vi "Rejestracja_konfiguracja.vi"(8 "error in (no error)":errorcluster, 11 "WolnaIn":T4={"WolnaStart"=FALSE, "WolnaPrzeglad"=FALSE, "Okres"=0.5, "Czas max"=120.0, "WolnaKonfiguracja"=FALSE, "Rej.1"={"Typ rejestracji"=enum."Wprost", "Kanały"=[1], "Opis"="Rej.X", "Aktywny"=FALSE, "Wolna Wykr num"=0}, "Rej.2"={"Typ rejestracji"=enum."Wprost", "Kanały"=[1], "Opis"="Rej.X", "Aktywny"=FALSE, "Wolna Wykr num"=0}, "Rej.3"={"Typ rejestracji"=enum."Wprost", "Kanały"=[1], "Opis"="Rej.X", "Aktywny"=FALSE, "Wolna Wykr num"=0}, "Rej.4"={"Typ rejestracji"=enum."Wprost", "Kanały"=[1], "Opis"="Rej.X", "Aktywny"=FALSE, "Wolna Wykr num"=0}, "Rej.5"={"Typ rejestracji"=enum."Wprost", "Kanały"=[1], "Opis"="Rej.X", "Aktywny"=FALSE, "Wolna Wykr num"=0}, "Rej.6"={"Typ rejestracji"=enum."Wprost", "Kanały"=[1], "Opis"="Rej.X", "Aktywny"=FALSE, "Wolna Wykr num"=0}, "Rej.7"={"Typ rejestracji"=enum."Wprost", "Kanały"=[1], "Opis"="Rej.X", "Aktywny"=FALSE, "Wolna Wykr num"=0}, "Rej.8"={"Typ rejestracji"=enum."Wprost", "Kanały"=[1], "Opis"="Rej.X", "Aktywny"=FALSE, "Wolna Wykr num"=0}} {"Rej.8"."Wolna Wykr num" items=["Brak", "Wykres 1", "Wykres 2", "Wykres 3", "Wykres 4"]; "Rej.7"."Wolna Wykr num" items=["Brak", "Wykres 1", "Wykres 2", "Wykres 3", "Wykres 4"]; "Rej.6"."Wolna Wykr num" items=["Brak", "Wykres 1", "Wykres 2", "Wykres 3", "Wykres 4"]; "Rej.5"."Wolna Wykr num" items=["Brak", "Wykres 1", "Wykres 2", "Wykres 3", "Wykres 4"]; "Rej.4"."Wolna Wykr num" items=["Brak", "Wykres 1", "Wykres 2", "Wykres 3", "Wykres 4"]; "Rej.3"."Wolna Wykr num" items=["Brak", "Wykres 1", "Wykres 2", "Wykres 3", "Wykres 4"]; "Rej.2"."Wolna Wykr num" items=["Brak", "Wykres 1", "Wykres 2", "Wykres 3", "Wykres 4"]; "Rej.1"."Wolna Wykr num" items=["Brak", "Wykres 1", "Wykres 2", "Wykres 3", "Wykres 4"]}) -> (0 "error out":errorcluster, 3 "WolnaOut":T4={"WolnaStart"=FALSE, "WolnaPrzeglad"=FALSE, "Okres"=0.5, "Czas max"=120.0, "WolnaKonfiguracja"=FALSE, "Rej.1"={"Typ rejestracji"=enum."Wprost", "Kanały"=[1], "Opis"="Rej.X", "Aktywny"=FALSE, "Wolna Wykr num"=0}, "Rej.2"={"Typ rejestracji"=enum."Wprost", "Kanały"=[1], "Opis"="Rej.X", "Aktywny"=FALSE, "Wolna Wykr num"=0}, "Rej.3"={"Typ rejestracji"=enum."Wprost", "Kanały"=[1], "Opis"="Rej.X", "Aktywny"=FALSE, "Wolna Wykr num"=0}, "Rej.4"={"Typ rejestracji"=enum."Wprost", "Kanały"=[1], "Opis"="Rej.X", "Aktywny"=FALSE, "Wolna Wykr num"=0}, "Rej.5"={"Typ rejestracji"=enum."Wprost", "Kanały"=[1], "Opis"="Rej.X", "Aktywny"=FALSE, "Wolna Wykr num"=0}, "Rej.6"={"Typ rejestracji"=enum."Wprost", "Kanały"=[1], "Opis"="Rej.X", "Aktywny"=FALSE, "Wolna Wykr num"=0}, "Rej.7"={"Typ rejestracji"=enum."Wprost", "Kanały"=[1], "Opis"="Rej.X", "Aktywny"=FALSE, "Wolna Wykr num"=0}, "Rej.8"={"Typ rejestracji"=enum."Wprost", "Kanały"=[1], "Opis"="Rej.X", "Aktywny"=FALSE, "Wolna Wykr num"=0}} {"Rej.8"."Wolna Wykr num" items=["Brak", "Wykres 1", "Wykres 2", "Wykres 3", "Wykres 4"]; "Rej.7"."Wolna Wykr num" items=["Brak", "Wykres 1", "Wykres 2", "Wykres 3", "Wykres 4"]; "Rej.6"."Wolna Wykr num" items=["Brak", "Wykres 1", "Wykres 2", "Wykres 3", "Wykres 4"]; "Rej.5"."Wolna Wykr num" items=["Brak", "Wykres 1", "Wykres 2", "Wykres 3", "Wykres 4"]; "Rej.4"."Wolna Wykr num" items=["Brak", "Wykres 1", "Wykres 2", "Wykres 3", "Wykres 4"]; "Rej.3"."Wolna Wykr num" items=["Brak", "Wykres 1", "Wykres 2", "Wykres 3", "Wykres 4"]; "Rej.2"."Wolna Wykr num" items=["Brak", "Wykres 1", "Wykres 2", "Wykres 3", "Wykres 4"]; "Rej.1"."Wolna Wykr num" items=["Brak", "Wykres 1", "Wykres 2", "Wykres 3", "Wykres 4"]})   [LabVIEW 2013]
uses:
  Kontrolki/GUI/Rejestracja_wolna.ctl
  Kontrolki/GUI/RejWol_konfig.ctl
  Kontrolki/GUI/RejWol_typ.ctl
  Kontrolki/GUI/Wolna_WykrNum.ctl
  Kontrolki/GUI/RejWol_konfig_opis.ctl
panel:
  out "appended path":path
  in  "Rejestracja 8":T1={"Typ rejestracji"=enum."Wprost", "Kanały"=[1], "Opis"="Rej.X", "Aktywny"=FALSE, "Wyświetlanie"=0} {"Wyświetlanie" items=["Brak", "Wykres 1", "Wykres 2", "Wykres 3", "Wykres 4"]; "Kanały" min=1 max=8}
  in  "Rejestracja 7":T1={"Typ rejestracji"=enum."Wprost", "Kanały"=[1], "Opis"="Rej.X", "Aktywny"=FALSE, "Wyświetlanie"=0} {"Wyświetlanie" items=["Brak", "Wykres 1", "Wykres 2", "Wykres 3", "Wykres 4"]; "Kanały" min=1 max=8}
  in  "Rejestracja 6":T1={"Typ rejestracji"=enum."Wprost", "Kanały"=[1], "Opis"="Rej.X", "Aktywny"=FALSE, "Wyświetlanie"=0} {"Wyświetlanie" items=["Brak", "Wykres 1", "Wykres 2", "Wykres 3", "Wykres 4"]; "Kanały" min=1 max=8}
  in  "Rejestracja 5":T1={"Typ rejestracji"=enum."Wprost", "Kanały"=[1], "Opis"="Rej.X", "Aktywny"=FALSE, "Wyświetlanie"=0} {"Wyświetlanie" items=["Brak", "Wykres 1", "Wykres 2", "Wykres 3", "Wykres 4"]; "Kanały" min=1 max=8}
  in  "Rejestracja 4":T1={"Typ rejestracji"=enum."Wprost", "Kanały"=[1], "Opis"="Rej.X", "Aktywny"=FALSE, "Wyświetlanie"=0} {"Wyświetlanie" items=["Brak", "Wykres 1", "Wykres 2", "Wykres 3", "Wykres 4"]; "Kanały" min=1 max=8}
  in  "Rejestracja 3":T1={"Typ rejestracji"=enum."Wprost", "Kanały"=[1], "Opis"="Rej.X", "Aktywny"=FALSE, "Wyświetlanie"=0} {"Wyświetlanie" items=["Brak", "Wykres 1", "Wykres 2", "Wykres 3", "Wykres 4"]; "Kanały" min=1 max=8}
  in  "Rejestracja 2":T1={"Typ rejestracji"=enum."Wprost", "Kanały"=[1], "Opis"="Rej.X", "Aktywny"=FALSE, "Wyświetlanie"=0} {"Wyświetlanie" items=["Brak", "Wykres 1", "Wykres 2", "Wykres 3", "Wykres 4"]; "Kanały" min=1 max=8}
  in  "Rejestracja 1":T1={"Typ rejestracji"=enum."Wprost", "Kanały"=[1], "Opis"="Rej.X", "Aktywny"=FALSE, "Wyświetlanie"=0} {"Wyświetlanie" items=["Brak", "Wykres 1", "Wykres 2", "Wykres 3", "Wykres 4"]; "Kanały" min=1 max=8}
  in  "Wczytaj":bool
  in  "Cancel Button":bool
  in  "OK Button":bool
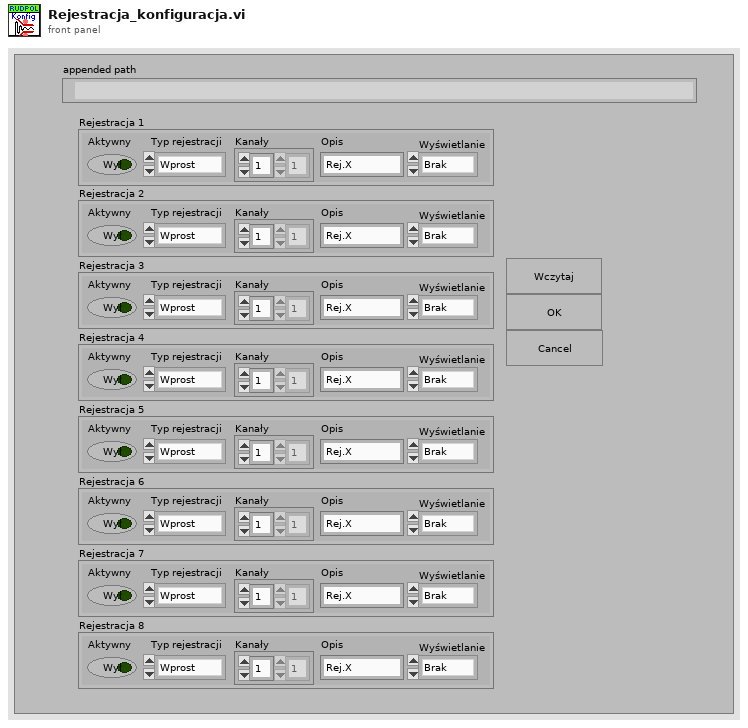
[diagram p1: front panel]
types:
  T1 = typedef "RejWol_konfig_opis.ctl" = cluster{"Typ rejestracji":T2, "Kanały":i32[], "Opis":string, "Aktywny":bool, "Wyświetlanie":T3}
  T2 = typedef "RejWol_typ.ctl" = enum16{"Wprost", "Moduł", "Kwadrat", "Iloczyn", "Faza"}
  T3 = typedef "Wolna_WykrNum.ctl" = u16
  T4 = typedef "Rejestracja_wolna.ctl" = cluster{"WolnaStart":bool, "WolnaPrzeglad":bool, "Okres":dbl, "Czas max":dbl, "WolnaKonfiguracja":bool, "Rej.1":T5, "Rej.2":T5, "Rej.3":T5, "Rej.4":T5, "Rej.5":T5, "Rej.6":T5, "Rej.7":T5, "Rej.8":T5}
  T5 = typedef "RejWol_konfig.ctl" = cluster{"Typ rejestracji":T2, "Kanały":i32[], "Opis":string, "Aktywny":bool, "Wolna Wykr num":T3}
  T6 = cluster{"Rej_konfig_out[0]":T5, "Rej_konfig_out[1]":T5, "Rej_konfig_out[2]":T5, "Rej_konfig_out[3]":T5, "Rej_konfig_out[4]":T5, "Rej_konfig_out[5]":T5, "Rej_konfig_out[6]":T5, "Rej_konfig_out[7]":T5, "Rej_konfig_out[8]":T5}
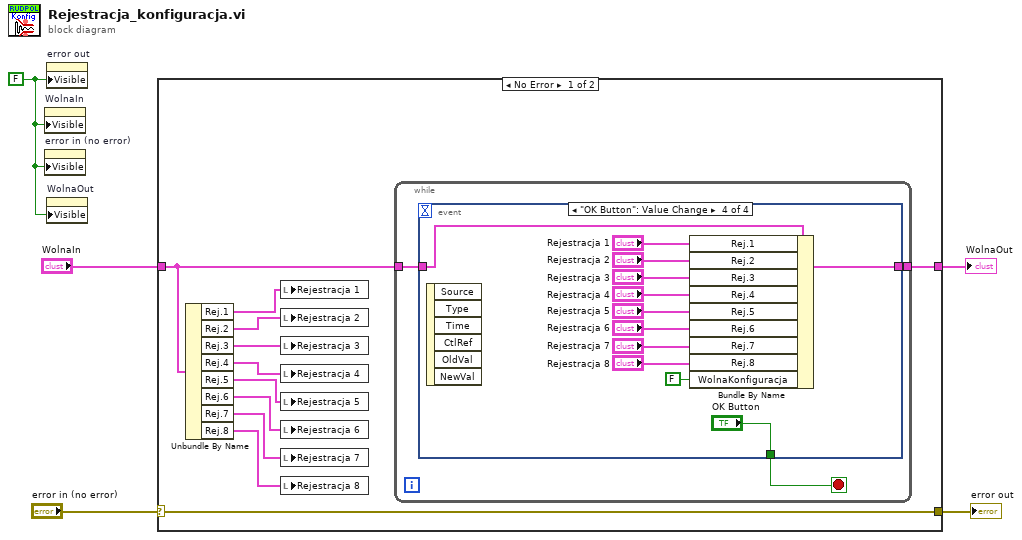
[diagram p0: block diagram]
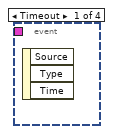
[diagram p2: hidden frame]
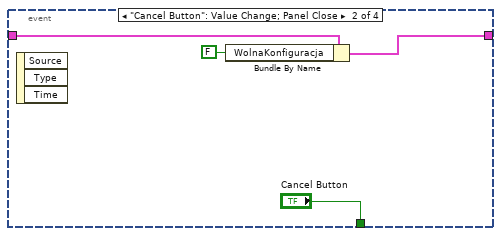
[diagram p3: hidden frame]
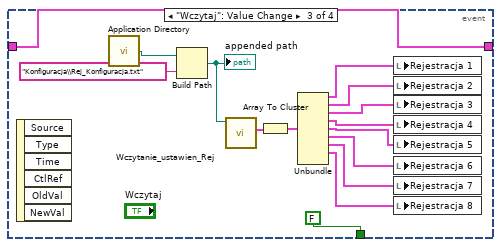
[diagram p4: hidden frame]
diagram:
  w2 = FALSE ("Visible")
  n1 = property on="WolnaIn" class="Clust (strict)"("Visible"=w2) -> ()  [unwired: 2 in, 2 out]
  n2 = property on="error in (no error)" class="Clust (strict)"("Visible"=w2) -> ()  [unwired: 2 in, 2 out]
  n3 = property on="error out" class="Clust (strict)"("Visible"=w2) -> ()  [unwired: 2 in, 2 out]
  n4 = property on="WolnaOut" class="Clust (strict)"("Visible"=w2) -> ()  [unwired: 2 in, 2 out]
  n5 = case shown="No Error" "error in (no error)" {
    selector: "error in (no error)" -> [w16 w52]
    tunnel: "WolnaIn" -> [w14 w51]
    tunnel: [w16 w52] -> w3
    tunnel: [w15 w51] -> w1
    frame No Error {
      n6 = Unbundle By Name(w14) -> ("Rej.1"=w6:T5, "Rej.2"=w13:T5, "Rej.3"=w12:T5, "Rej.4"=w11:T5, "Rej.5"=w10:T5, "Rej.6"=w9:T5, "Rej.7"=w8:T5, "Rej.8"=w7:T5)
      n7 = local write "Rejestracja 1"(w6) -> ()
      n8 = local write "Rejestracja 2"(w13) -> ()
      n9 = local write "Rejestracja 3"(w12) -> ()
      n10 = local write "Rejestracja 4"(w11) -> ()
      n11 = local write "Rejestracja 5"(w10) -> ()
      n12 = local write "Rejestracja 6"(w9) -> ()
      n13 = local write "Rejestracja 7"(w8) -> ()
      n14 = local write "Rejestracja 8"(w7) -> ()
      n15 = while {
        tunnel: w14 -> [w18]
        tunnel: [w17] -> w15
        stop <- w19 stop-if-true
        n16 = event shown="[3] \"OK Button\": Value Change" {
          selector: _ -> [_ _ _ _]
          dyn-events: _ -> [_ _ _ _]
          timeout: _ -> [_ _ _ _]
          tunnel: [_ "Cancel Button" FALSE ("OK Button") "OK Button"] -> w19
          tunnel: w18 -> [_ w22 w36 w49]
          tunnel: [_ w21 w36 w48] -> w17
          event Timeout {
            n17 = event-data() -> ()  [unwired: 1 in, 3 out]
          }
          event "Cancel Button": Value Change; Panel Close {
            n18 = event-data() -> ()  [unwired: 1 in, 3 out]
            n19 = Bundle By Name(cluster=w22, "WolnaKonfiguracja"=FALSE) -> (w21:T4)
          }
          event "Wczytaj": Value Change {
            n20 = event-data() -> ()  [unwired: 1 in, 6 out]
            n21 = call <vilib>:"Application Directory.vi"() -> ("Application Directory"=w24:path)
            n22 = Build Path(base path=w24, name or relative path="Konfiguracja\\Rej_Konfiguracja.txt") -> (appended path=w35:path)
            "appended path" <- w35
            n23 = call "Wczytanie_ustawien_Rej.vi"("Plik konf in"=w35) -> ("Rej_konfig_out"=w34:T5[])  [unwired: 8 in, 2 out]
            n24 = Array To Cluster(array=w34) -> (cluster=w33:T6)
            n25 = Unbundle(w33) -> ("Rej_konfig_out[0]"=w32:T5, "Rej_konfig_out[1]"=w31:T5, "Rej_konfig_out[2]"=w30:T5, "Rej_konfig_out[3]"=w29:T5, "Rej_konfig_out[4]"=w28:T5, "Rej_konfig_out[5]"=w27:T5, "Rej_konfig_out[6]"=w26:T5, "Rej_konfig_out[7]"=w25:T5)  [unwired: 1 out]
            n26 = local write "Rejestracja 1"(w32) -> ()
            n27 = local write "Rejestracja 2"(w31) -> ()
            n28 = local write "Rejestracja 3"(w30) -> ()
            n29 = local write "Rejestracja 4"(w29) -> ()
            n30 = local write "Rejestracja 5"(w28) -> ()
            n31 = local write "Rejestracja 6"(w27) -> ()
            n32 = local write "Rejestracja 7"(w26) -> ()
            n33 = local write "Rejestracja 8"(w25) -> ()
          }
          event "OK Button": Value Change {
            n34 = event-data() -> ()  [unwired: 1 in, 6 out]
            n35 = Bundle By Name(cluster=w49, "Rej.1"="Rejestracja 1", "Rej.2"="Rejestracja 2", "Rej.3"="Rejestracja 3", "Rej.4"="Rejestracja 4", "Rej.5"="Rejestracja 5", "Rej.6"="Rejestracja 6", "Rej.7"="Rejestracja 7", "Rej.8"="Rejestracja 8", "WolnaKonfiguracja"=FALSE) -> (w48:T4)
          }
        }
      }
    }
    frame Error {
    }
  }
  "WolnaOut" <- w1
  "error out" <- w3
